vi "TestHelper_RandI32.vi"(10 "Min":i32, 11 "Max":i32=10) -> (2 "Rand i32":i32)   [LabVIEW 2017]
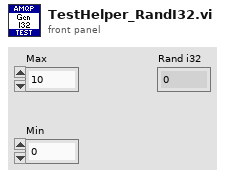
[diagram p1: front panel]
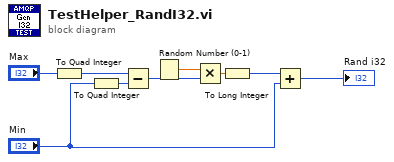
[diagram p0: block diagram]
diagram:
  n1 = To Quad Integer(1:"Max") -> (0:w3:i64)
  n2 = To Quad Integer(1:"Min") -> (0:w2:i64)
  n3 = Subtract(x=w3, y=w2) -> (x-y=w6:i64)
  n4 = Random Number (0-1)() -> (number: 0 to 1=w7:dbl)
  n5 = Multiply(x=w7, y=w6) -> (x*y=w8:dbl)
  n6 = To Long Integer(number=w8) -> (32bit integer=w5:i32)
  n7 = Add(x=w5, y="Min") -> (x+y=→"Rand i32":i32)
